vi "AlgorithmOptimizeXYPLOT.vi"(2 "MatchBallY":dbl, 3 "MatchBallX":dbl, 4 "D2 Y COM":dbl, 5 "D2 X COM":dbl, 6 "D1Y COM":dbl, 7 "D1 X COM 2":dbl) -> (0 "Plot":T1, 1 "THETA":dbl)   [LabVIEW 2014]
panel:
  out "Angles":dbl[](array[numeric])
  out "max index(es)":i32
  out "max value":dbl
  out "Minimum X separations":dbl[](array[numeric])
  # "theta Calculation"
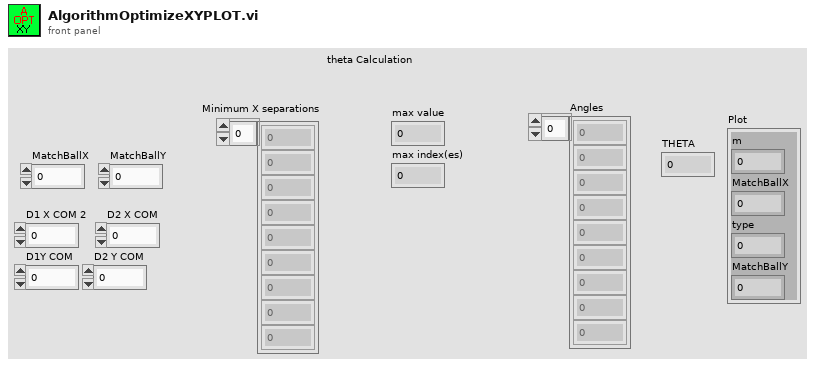
[diagram p1: front panel]
types:
  T1 = cluster{"m":dbl, "MatchBallX":dbl, "type":dbl, "MatchBallY":dbl}
  T2 = cluster{"kLW":dbl, "CoLW":dbl, "type":dbl, "dummy":dbl}
  T3 = cluster{"m":dbl, "MatchBallX":dbl, "type":dbl, "MatchBallY":dbl}[]
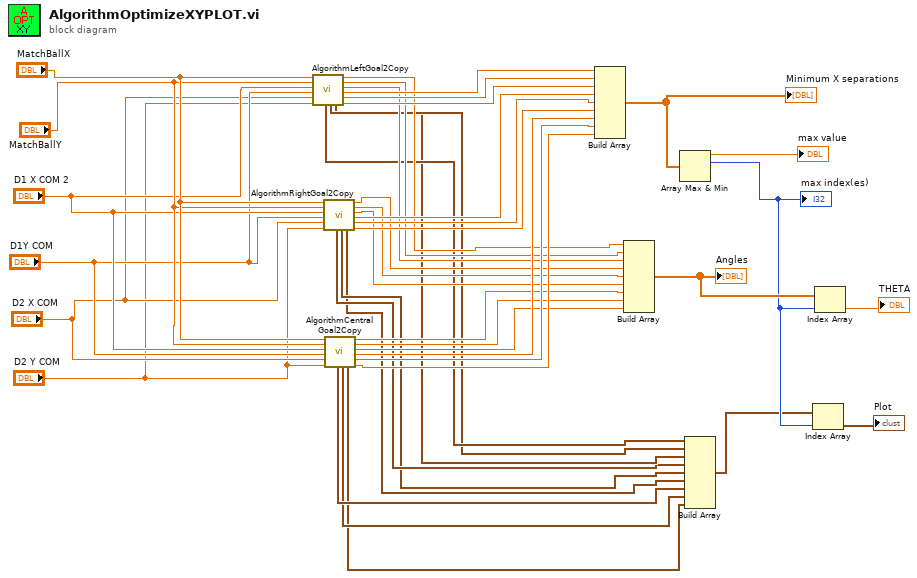
[diagram p0: block diagram]
diagram:
  n1 = call "AlgorithmLeftGoal2Copy.vi"("MatchBallX"="MatchBallX", "MatchBallY"="MatchBallY", "D1 X COM"="D1 X COM 2", "D1Y COM"="D1Y COM", "D2 X COM"="D2 X COM", "D2 Y COM"="D2 Y COM") -> ("LW"=w11:T2, "RW"=w10:cluster{"kRW":dbl, "CoRW":dbl, "y":dbl, "y":dbl}, "output cluster"=w9:T1, "Theta LG,LW"=w25:dbl, "aRW"=w24:dbl, "aS"=w23:dbl, "min x"=w34:dbl, "min x2"=w33:dbl, "min x3"=w32:dbl)  [unwired: 5 in]
  n2 = call "AlgorithmRightGoal2Copy.vi"("MatchBallX"="MatchBallX", "MatchBallY"="MatchBallY", "D1 X COM"="D1 X COM 2", "D1Y COM"="D1Y COM", "D2 X COM"="D2 X COM", "D2 Y COM"="D2 Y COM") -> ("LW"=w8:cluster{"kLW":dbl, "CoLW":dbl, "y":dbl, "y":dbl}, "RW"=w7:cluster{"kRW":dbl, "CoRW":dbl, "y":dbl, "y":dbl}, "output cluster"=w6:T1, "Theta LG,LW"=w22:dbl, "aRW"=w21:dbl, "aS"=w20:dbl, "min x"=w31:dbl, "min x2"=w30:dbl, "min x3"=w29:dbl)  [unwired: 5 in]
  n3 = call "AlgorithmCentralGoal2Copy.vi"("MatchBallX"="MatchBallX", "MatchBallY"="MatchBallY", "D1 X COM"="D1 X COM 2", "D1Y COM"="D1Y COM", "D2 X COM"="D2 X COM", "D2 Y COM"="D2 Y COM") -> ("LW"=w4:cluster{"kLW":dbl, "CoLW":dbl, "y":dbl, "y":dbl}, "RW"=w3:cluster{"kRW":dbl, "CoRW":dbl, "y":dbl, "y":dbl}, "output cluster"=w2:T1, "Theta LG,LW"=w19:dbl, "aRW"=w18:dbl, "aS"=w17:dbl, "min x"=w28:dbl, "min x2"=w27:dbl, "min x3"=w26:dbl)  [unwired: 5 in]
  n4 = Build Array(w34, w33, w32, w31, w30, w29, w28, w27, w26) -> (w16:dbl[])
  "Minimum X separations" <- w16
  n5 = Build Array(w25, w24, w23, w22, w21, w20, w19, w18, w17) -> (w14:dbl[])
  "Angles" <- w14
  n6 = Array Max & Min(array=w16) -> (max value=→"max value":dbl, max index (indices)=w12:i32)  [unwired: 2 out]
  "max index(es)" <- w12
  n7 = Build Array(w11, w10, w9, w8, w7, w6, w4, w3, w2) -> (w5:T3)
  n8 = Index Array(array=w5, index=w12) -> (element=→"Plot":T1)
  n9 = Index Array(array=w14, index=w12) -> (element=→"THETA":dbl)
